vi "Get Sub Waveform.vi"(8 "error in (no error)":errorcluster, 10 "index":i32, 11 "Composite Waveform in":refnum<class "Composite Waveform.lvclass">) -> (0 "error out":errorcluster, 2 "Waveform.lvclass":refnum<class "Waveform.lvclass">, 3 "Composite Waveform out":refnum<class "Composite Waveform.lvclass">)   [LabVIEW 2016, in "Composite Waveform.lvclass"]
uses:
  Composite Waveform.lvclass
  Waveform/Waveform.lvclass
  Composite Waveform.lvclass/Composite Waveform.ctl
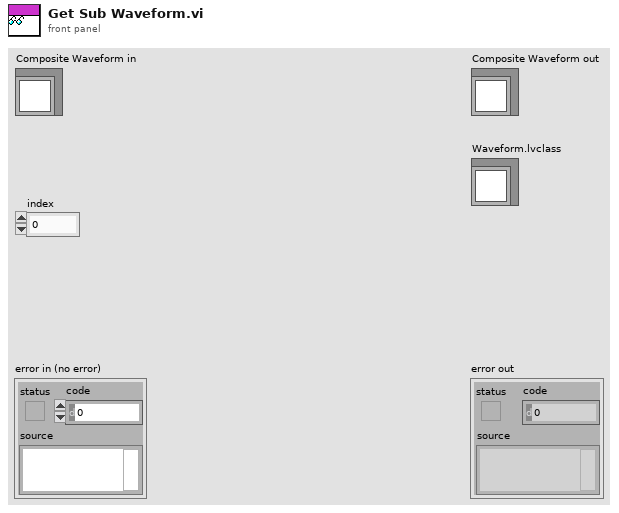
[diagram p1: front panel]
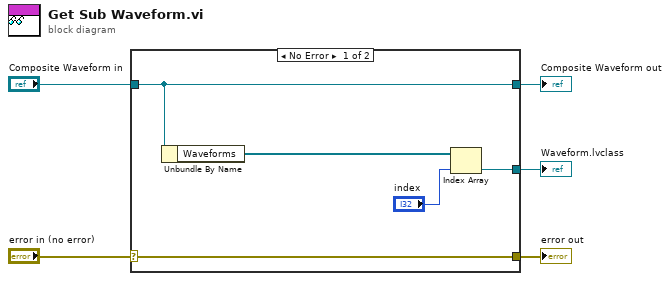
[diagram p0: block diagram]
diagram:
  n1 = case shown="No Error" "error in (no error)" {
    selector: "error in (no error)" -> [w10 w11]
    tunnel: [w10 w11] -> w4
    tunnel: [w9 w12] -> w2
    tunnel: "Composite Waveform in" -> [w9 w12]
    tunnel: [w6 _] -> w1
    frame No Error {
      n2 = Unbundle By Name(w9) -> ("Waveforms"=w8:refnum<class "Waveform.lvclass">[])
      n3 = Index Array(array=w8, index="index") -> (element=w6:refnum<class "Waveform.lvclass">)
    }
    frame Error {
    }
  }
  "error out" <- w4
  "Composite Waveform out" <- w2
  "Waveform.lvclass" <- w1
